vi "Calculate-I_T.vi"() -> ()   [LabVIEW 2023]
panel:
  out "L":dbl
  in  "desired tip-to-substrate distance / um":dbl
  out "area of UME / um2":dbl
  out "radius / um":dbl
  in  "i_ss (nA)":dbl
  out "Concentration / mol/cm3":dbl
  in  "K3Fe(CN)6 / g":dbl
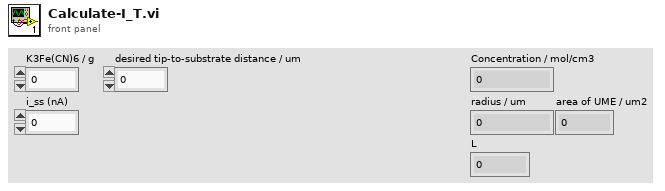
[diagram p1: front panel]
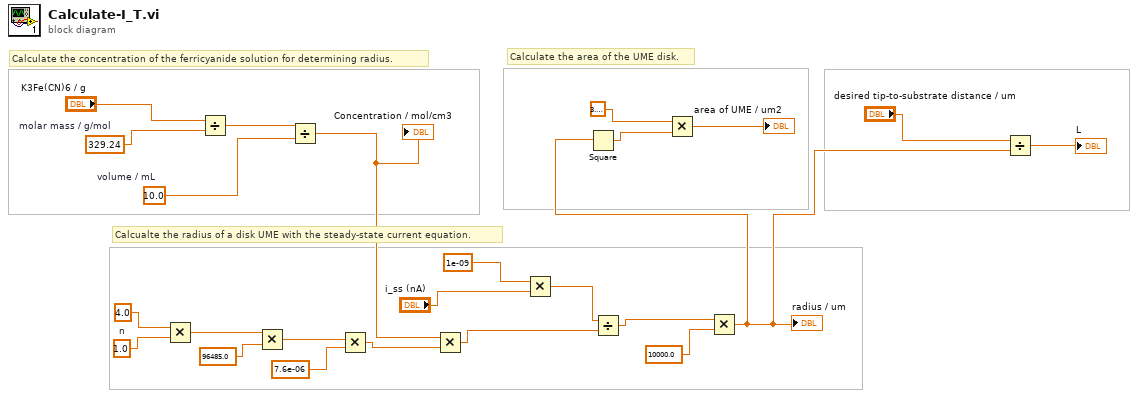
[diagram p0: block diagram]
diagram:
  w19 = 1.0  # n
  w22 = 329.24  # molar mass / g/mol
  w24 = 10.0  # volume / mL
  # "Calculate the area of the UME disk."
  # "Calcualte the radius of a disk UME with the steady-state current equation."
  # "Calculate the concentration of the ferricyanide solution for determining radius."
  n1 = Multiply(x=4.0, y=w19) -> (x*y=w18:dbl)
  n2 = Divide(x="K3Fe(CN)6 / g", y=w22) -> (x/y=w21:dbl)
  n3 = Multiply(x=w18, y=96485.0) -> (x*y=w16:dbl)
  n4 = Divide(x=w21, y=w24) -> (x/y=w14:dbl)
  "Concentration / mol/cm3" <- w14
  n5 = Multiply(x=w16, y=7.6e-06) -> (x*y=w13:dbl)
  n6 = Multiply(x=w14, y=w13) -> (x*y=w9:dbl)
  n7 = Multiply(x=1e-09, y="i_ss (nA)") -> (x*y=w10:dbl)
  n8 = Divide(x=w10, y=w9) -> (x/y=w7:dbl)
  n9 = Multiply(x=w7, y=10000.0) -> (x*y=w1:dbl)
  "radius / um" <- w1
  n10 = Square(x=w1) -> (x^2=w6:dbl)
  n11 = Multiply(x=3.141592653589793, y=w6) -> (x*y=→"area of UME / um2":dbl)
  n12 = Divide(x="desired tip-to-substrate distance / um", y=w1) -> (x/y=→"L":dbl)
